vi "EnergyControlling.vi"() -> ()   [LabVIEW 2017]
uses:
  classes/DataCollector.lvclass
  classes/DataHandler.lvclass
  classes/SimulationParameter.lvclass
panel:
  in  "Controlling":T1={"Prioritization"=0, "Operating Mode"="", "Release Time "={"Start"=0.0, "Stop"=0.0}, "Activity"=TRUE, " Limitation"={"El. Power"=0.0, "Th. Power"=0.0}}
  in  "Field Elements":i32(listbox)
  in  "Management-Typs":u16(ring) items=["ManagementRandomData.vi", "ManagementRandomData2.vi"]
  in  "Stop":bool
  out "Control-Matrix-Overview":i32(listbox)=-1
  in  "application reference (local)":refnum<vi>
  out "Array":path[](array[path])
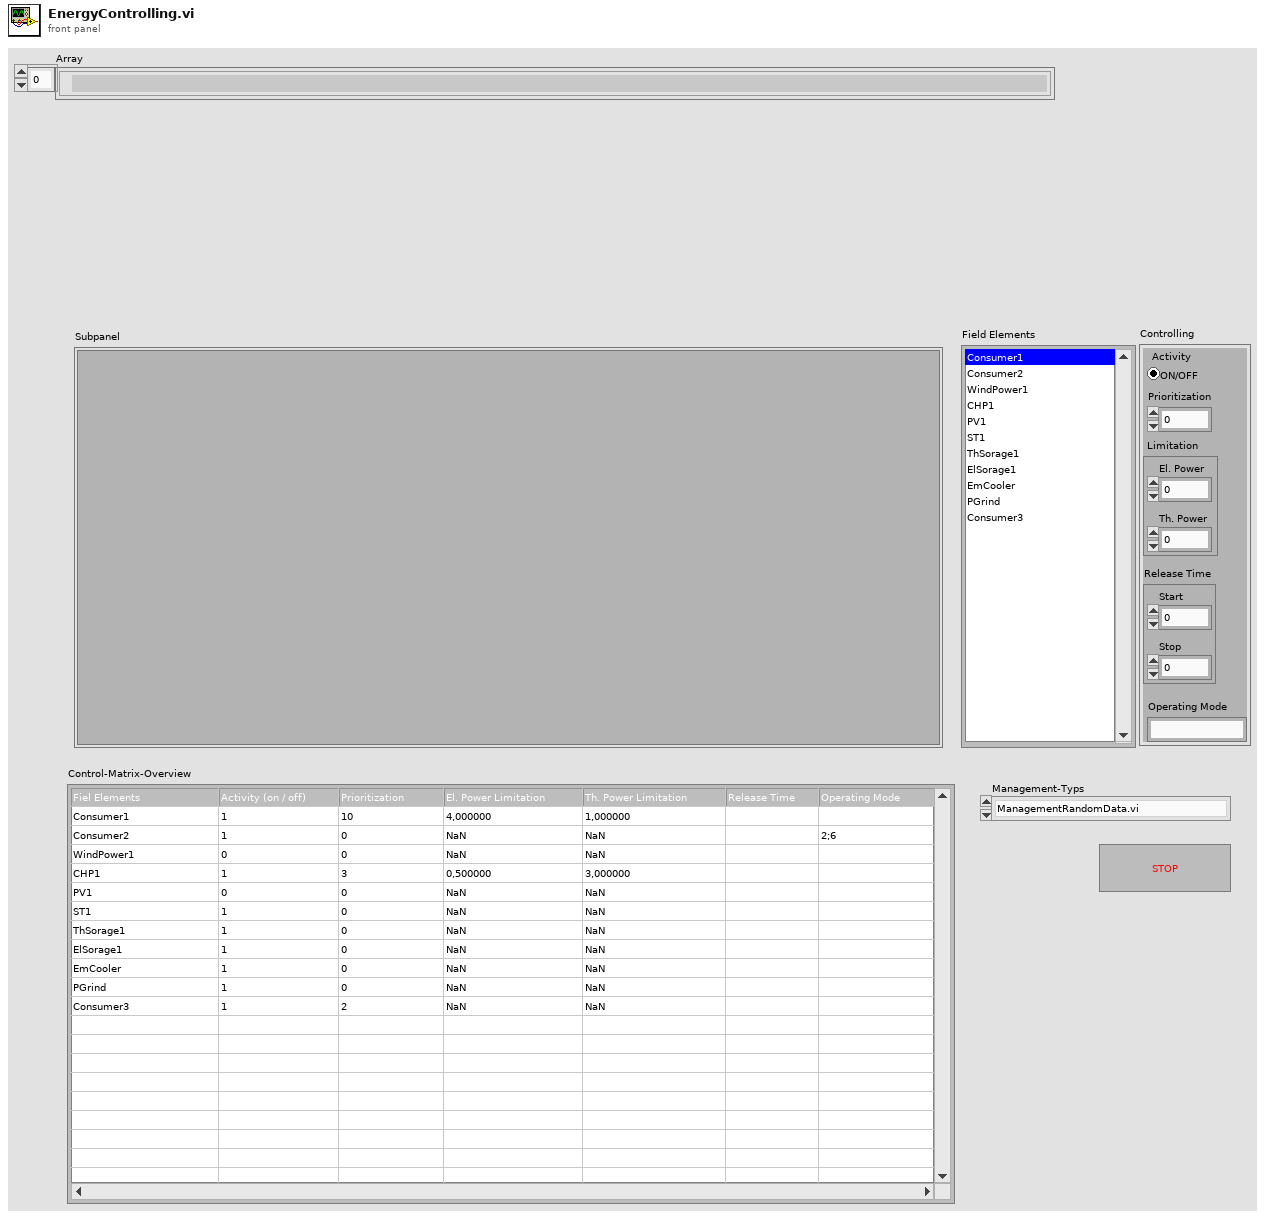
[diagram p1: front panel]
types:
  T1 = cluster{"Prioritization":i8, "Operating Mode":string, "Release Time ":cluster{"Start":dbl, "Stop":dbl}, "Activity":bool, " Limitation":cluster{"El. Power":dbl, "Th. Power":dbl}}
  T2 = cluster{"DataCollector out":refnum<class "DataCollector.lvclass">, "DataHandler out":refnum<class "DataHandler.lvclass">}
  T3 = cluster{"DataCollector":refnum<class "DataCollector.lvclass">, "DataHandling":refnum<class "DataHandler.lvclass">, "SimulationParameter":refnum<class "SimulationParameter.lvclass">}
  T4 = cluster{"DataCollector":refnum<class "DataCollector.lvclass">, "DataHandling":refnum<class "DataHandler.lvclass">}
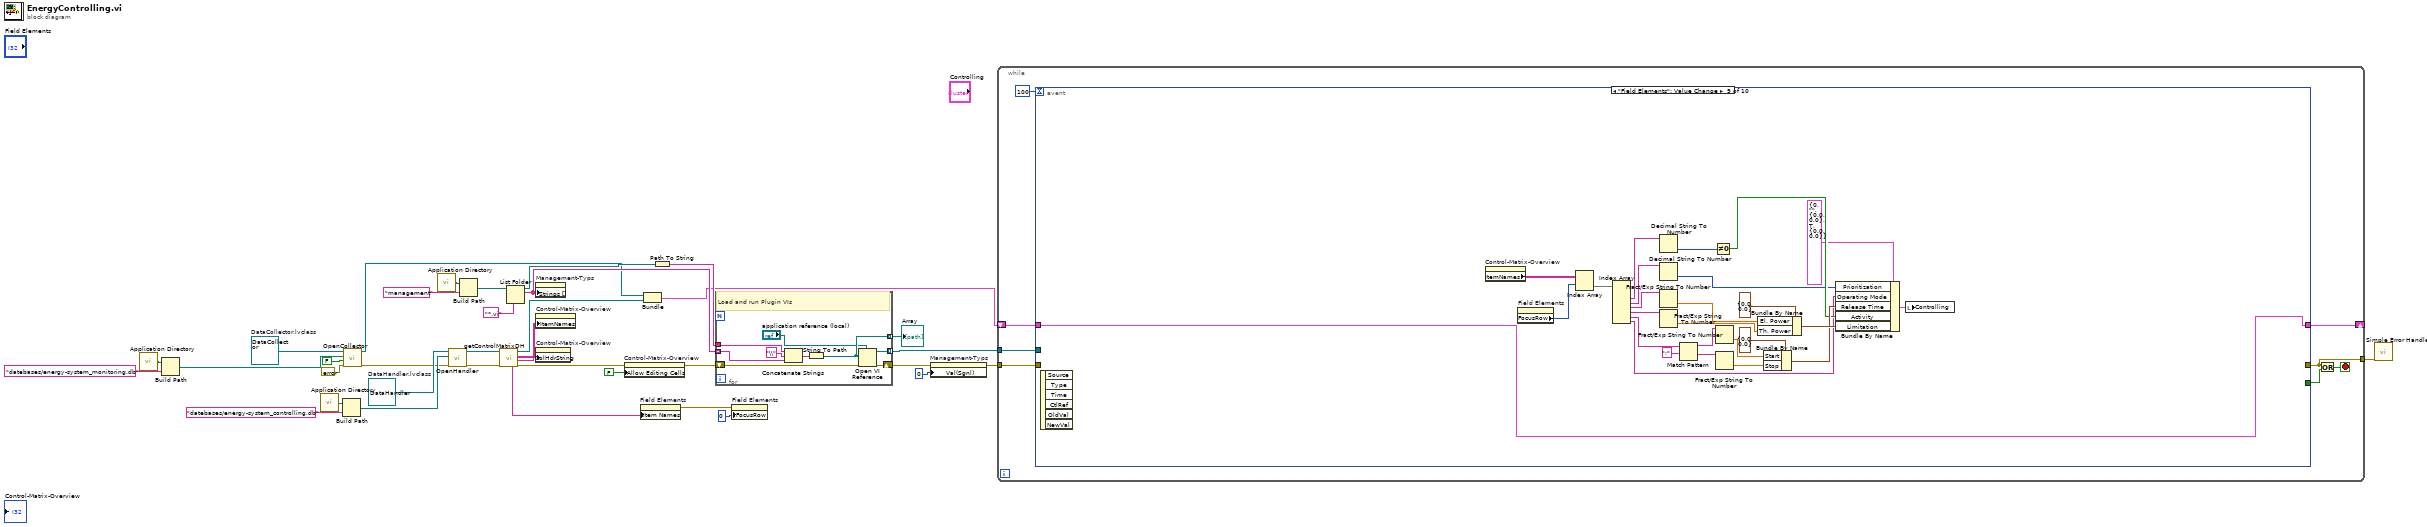
[diagram p0: block diagram]
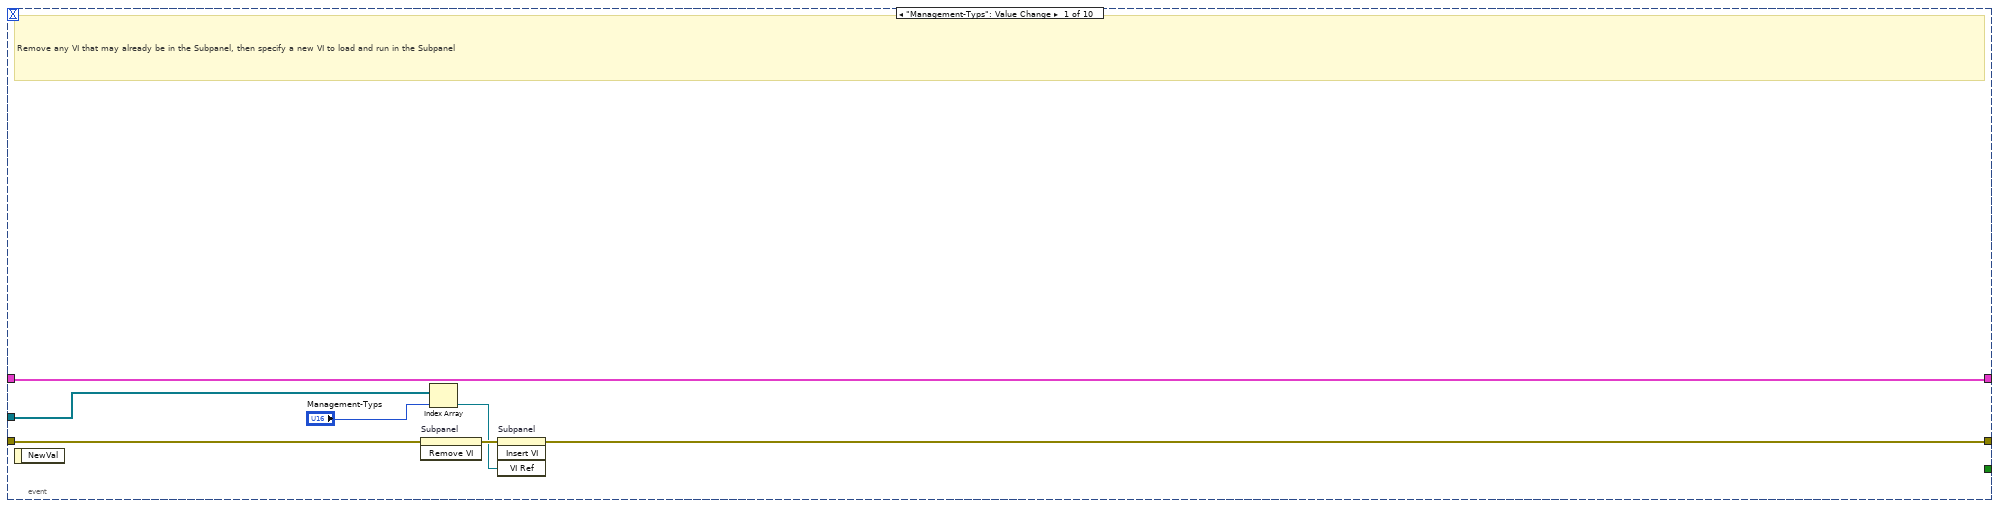
[diagram p2: hidden frame]
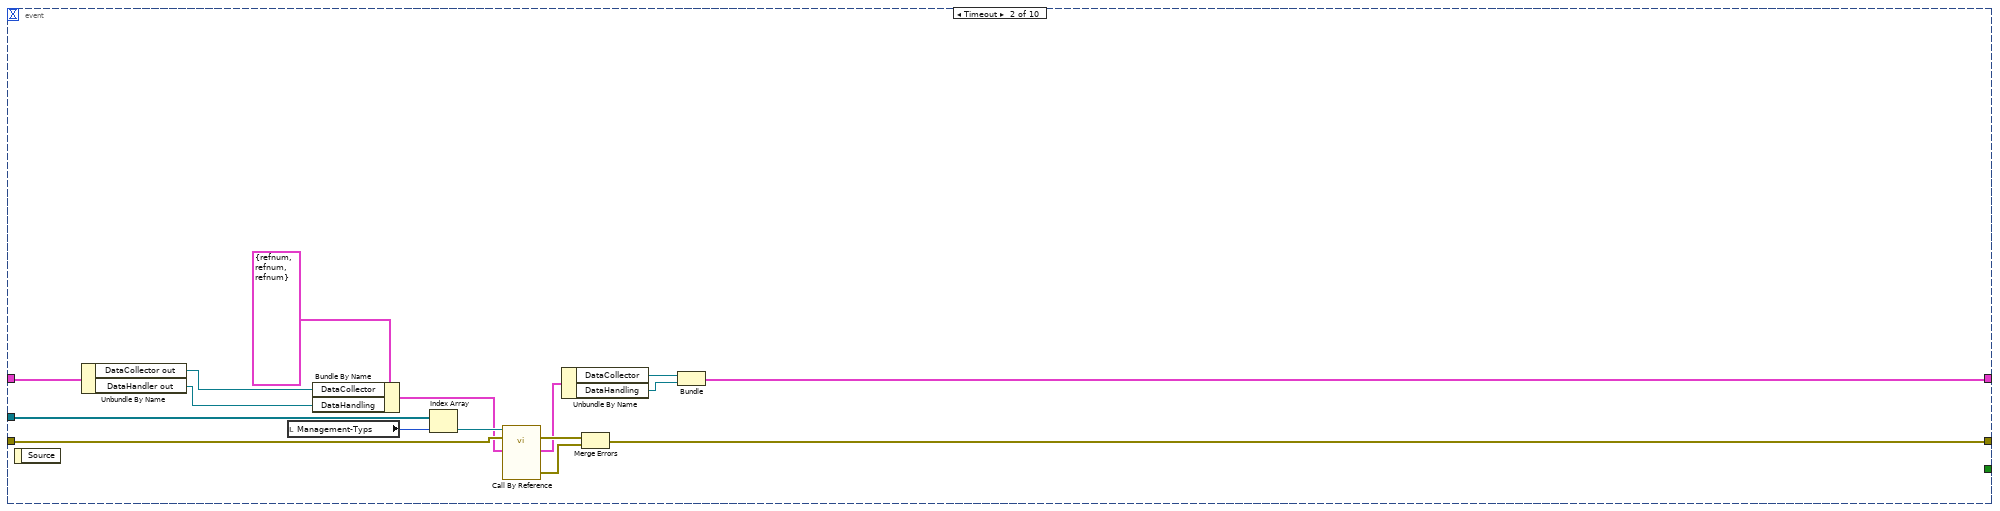
[diagram p3: hidden frame]
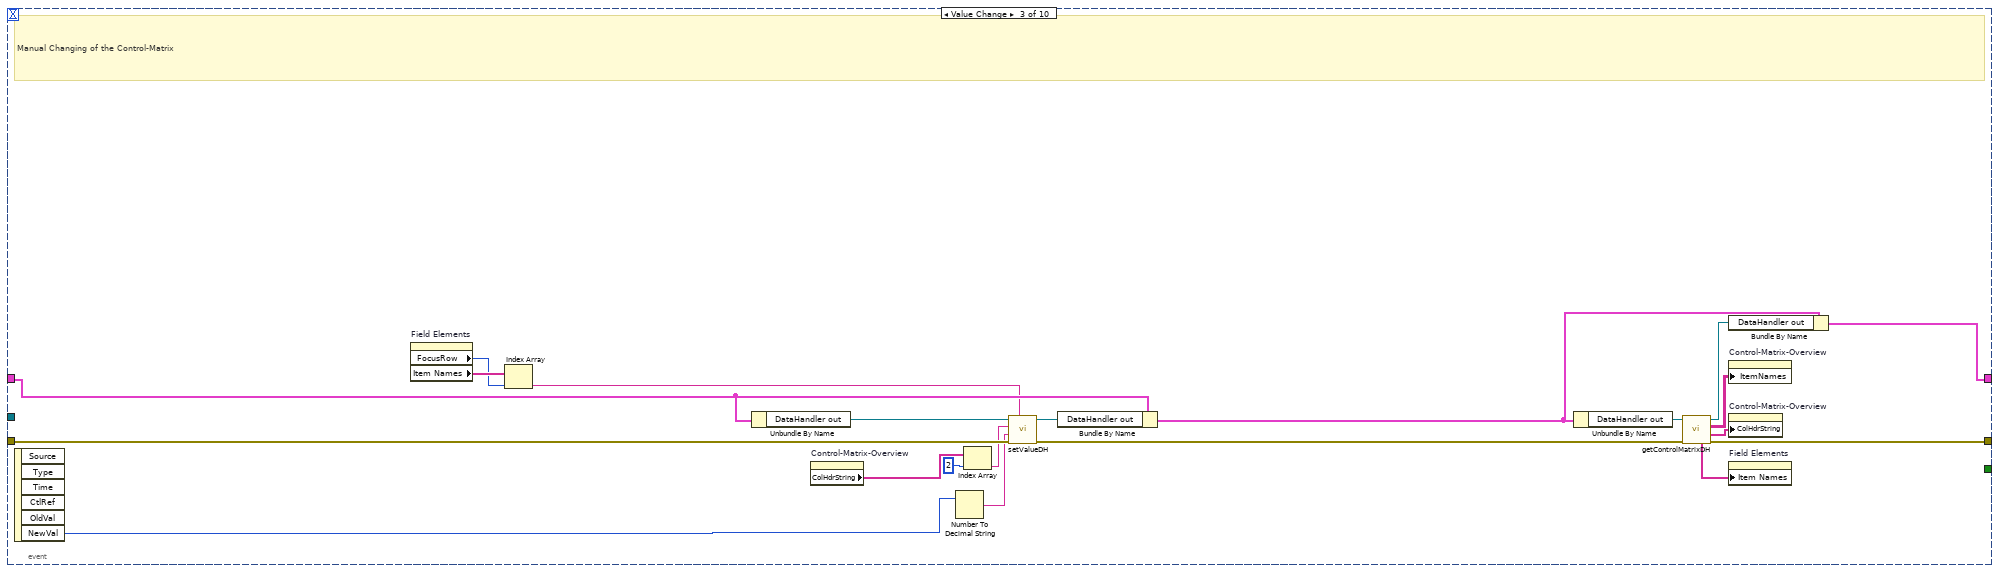
[diagram p4: hidden frame]
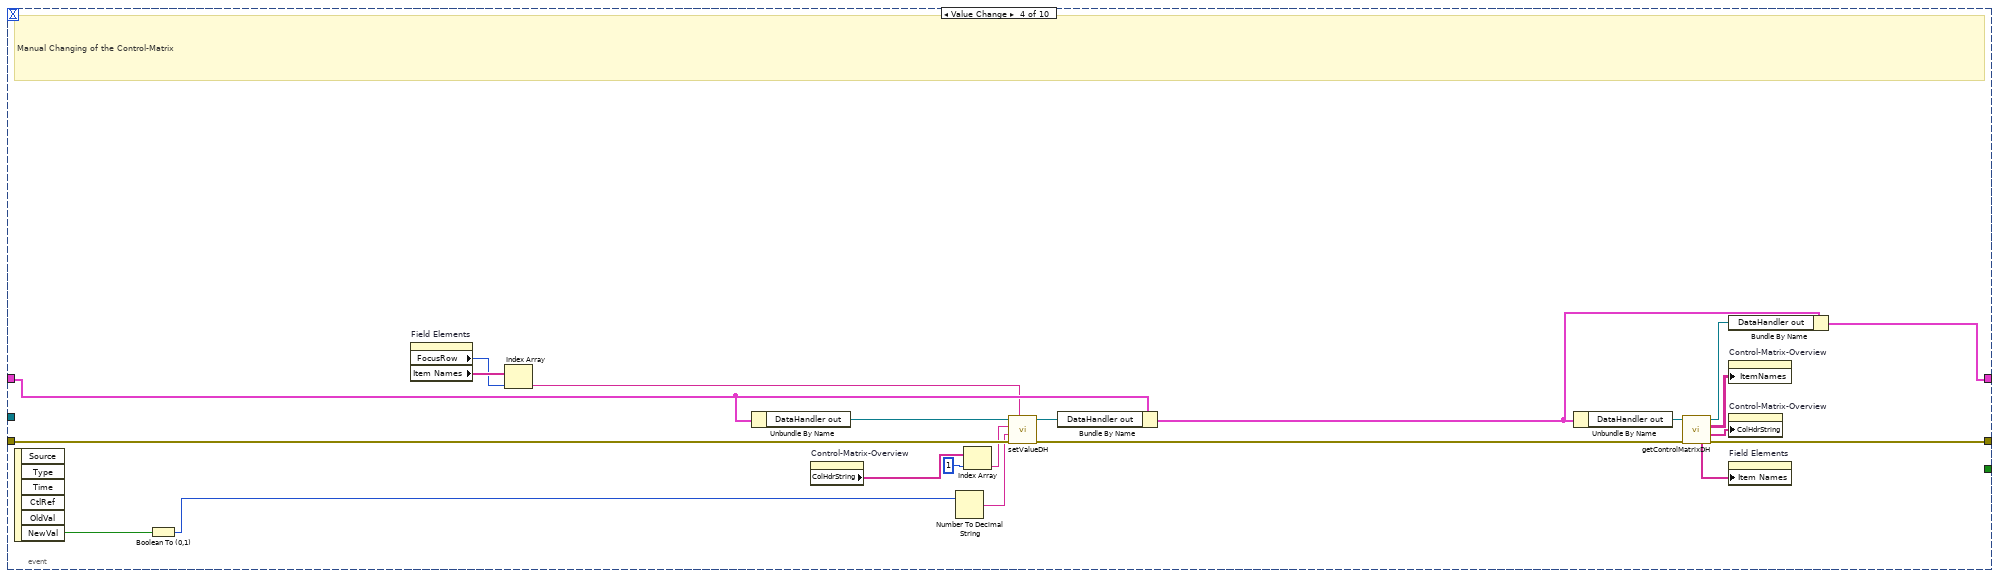
[diagram p5: hidden frame]
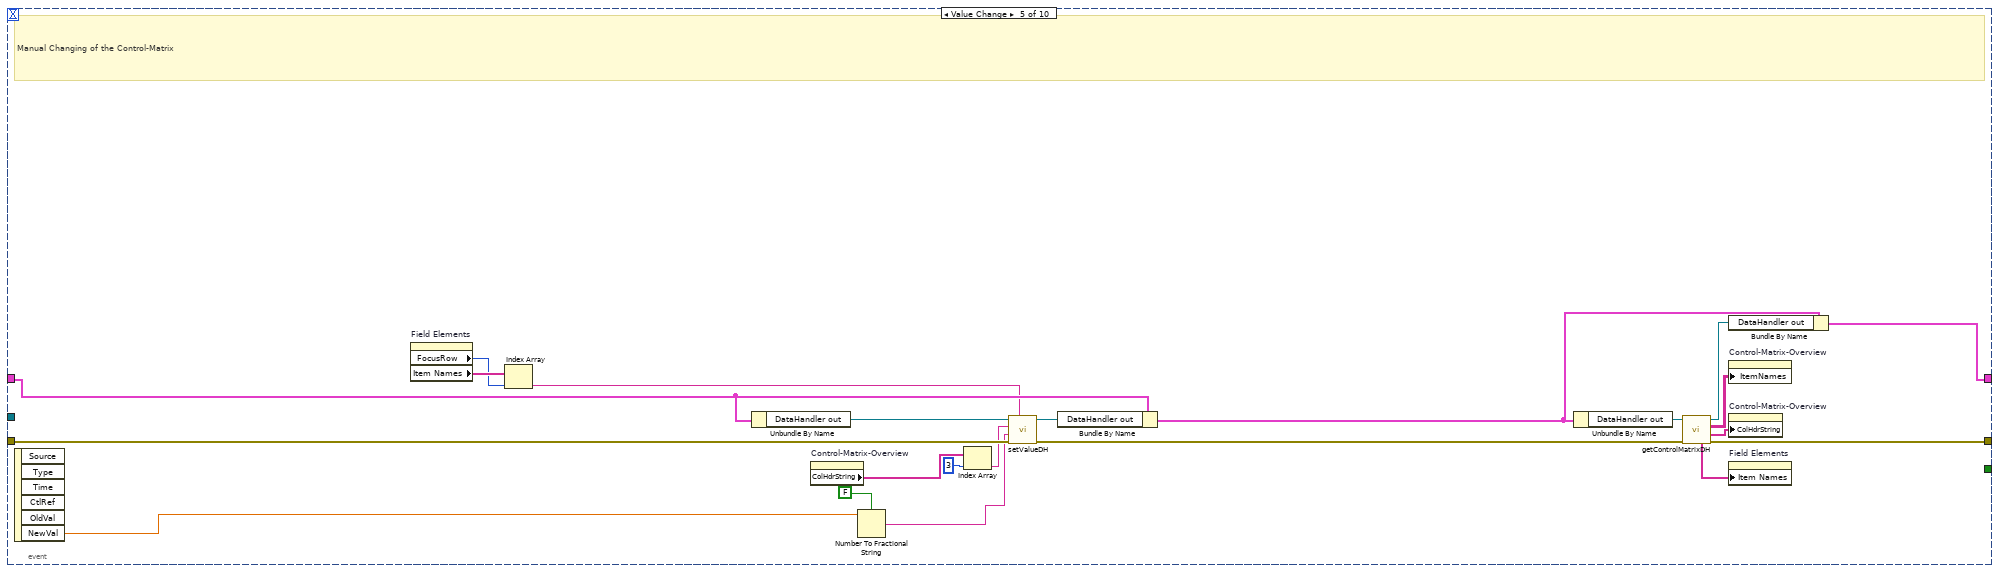
[diagram p6: hidden frame]
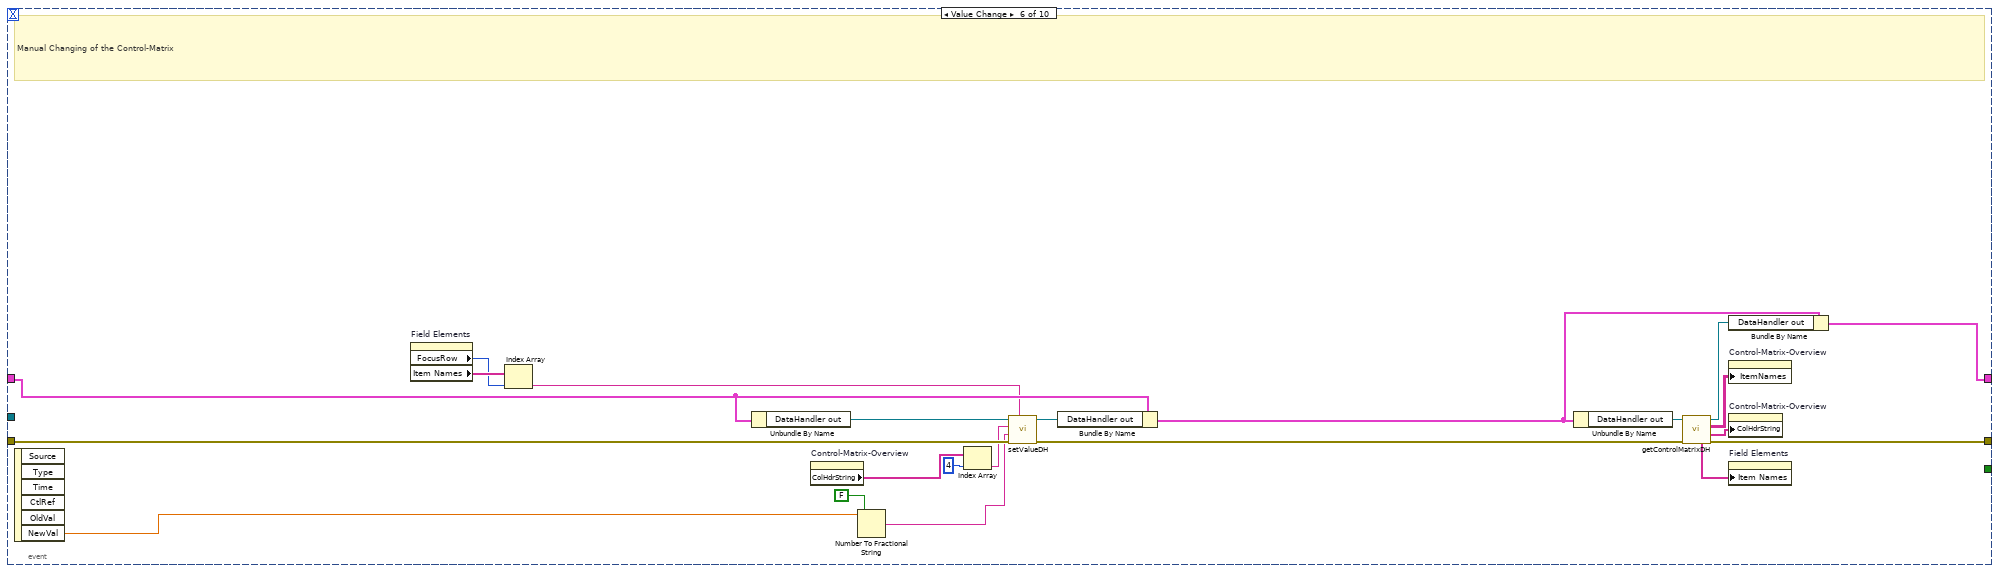
[diagram p7: hidden frame]
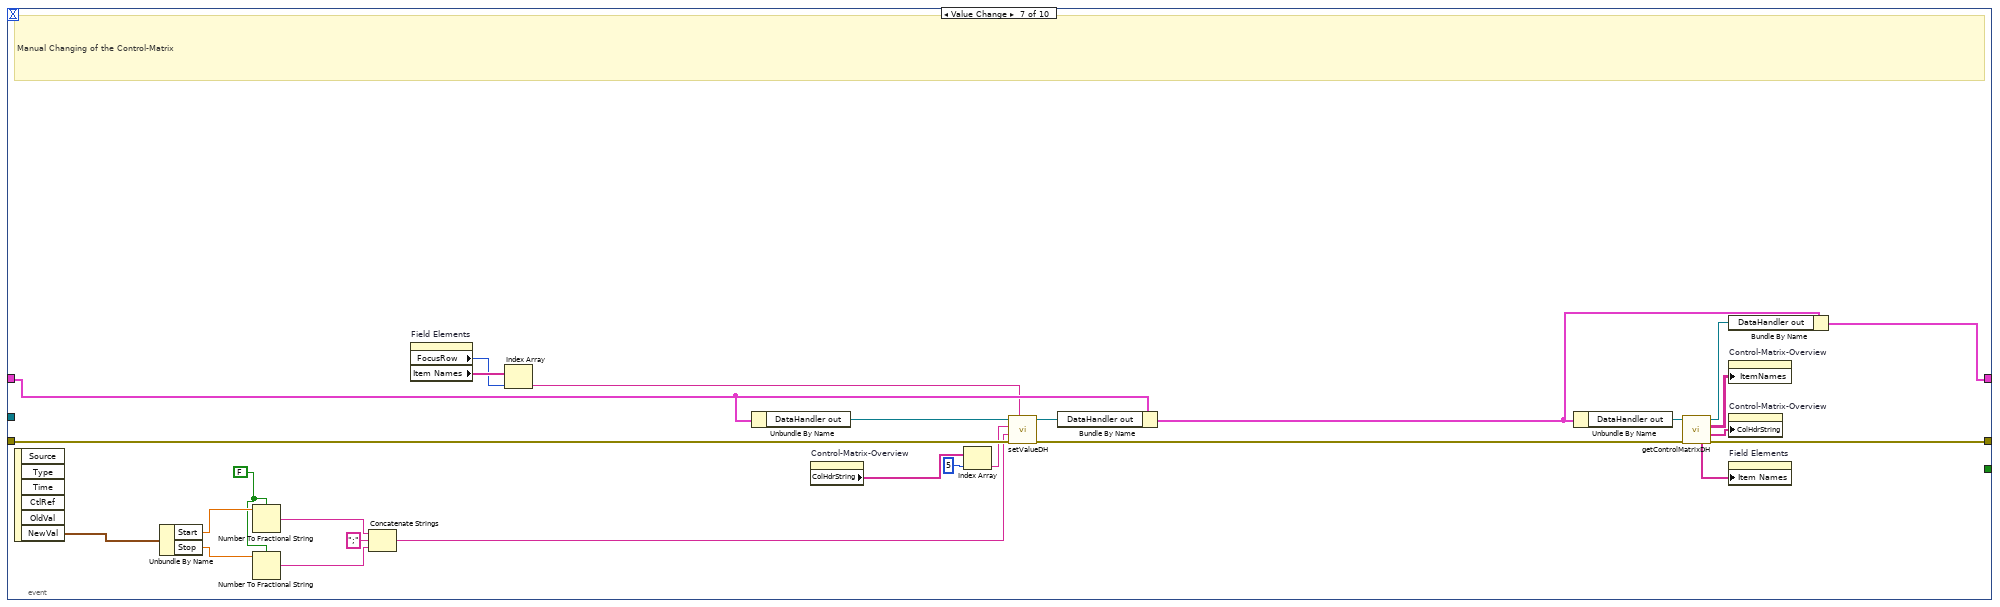
[diagram p8: hidden frame]
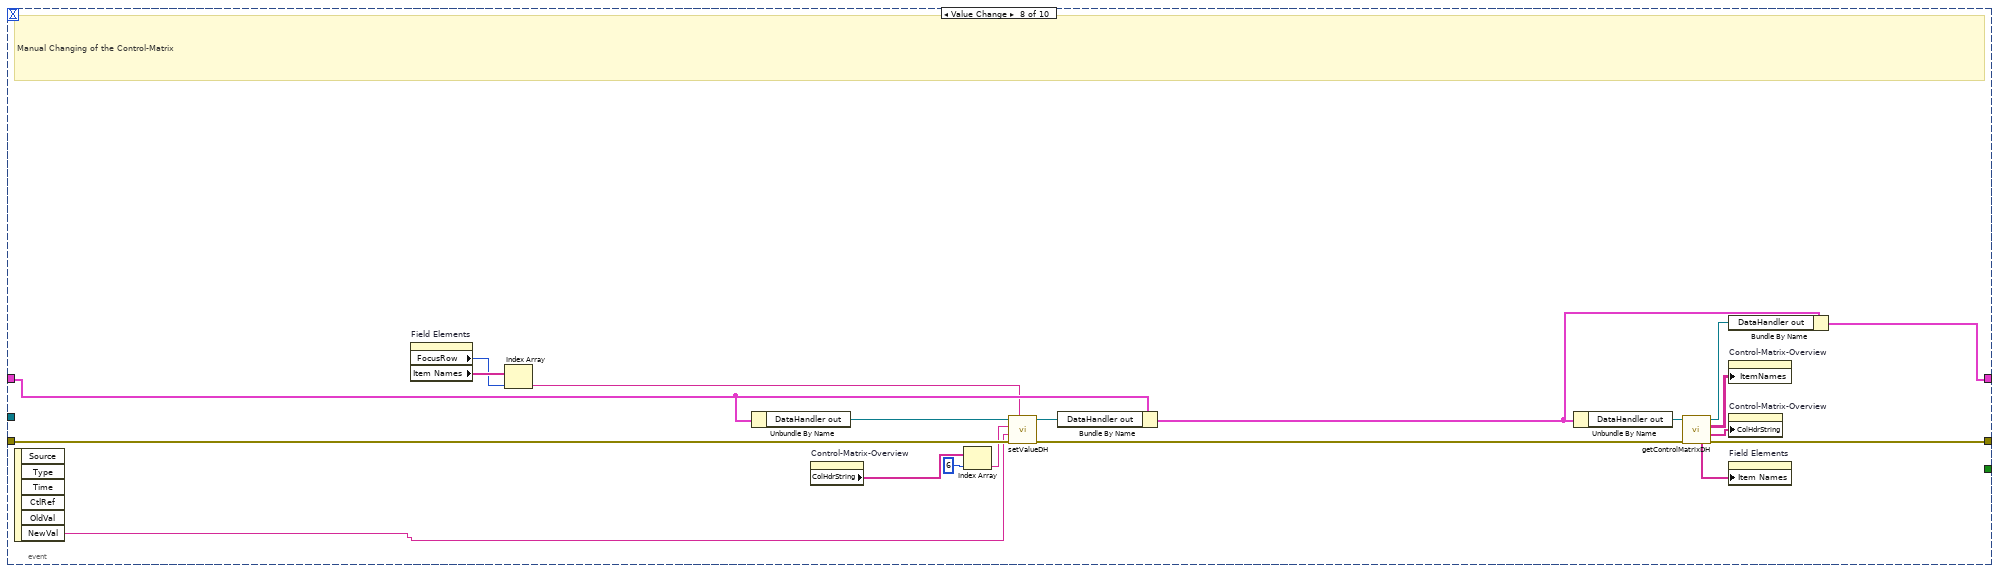
[diagram p9: hidden frame]
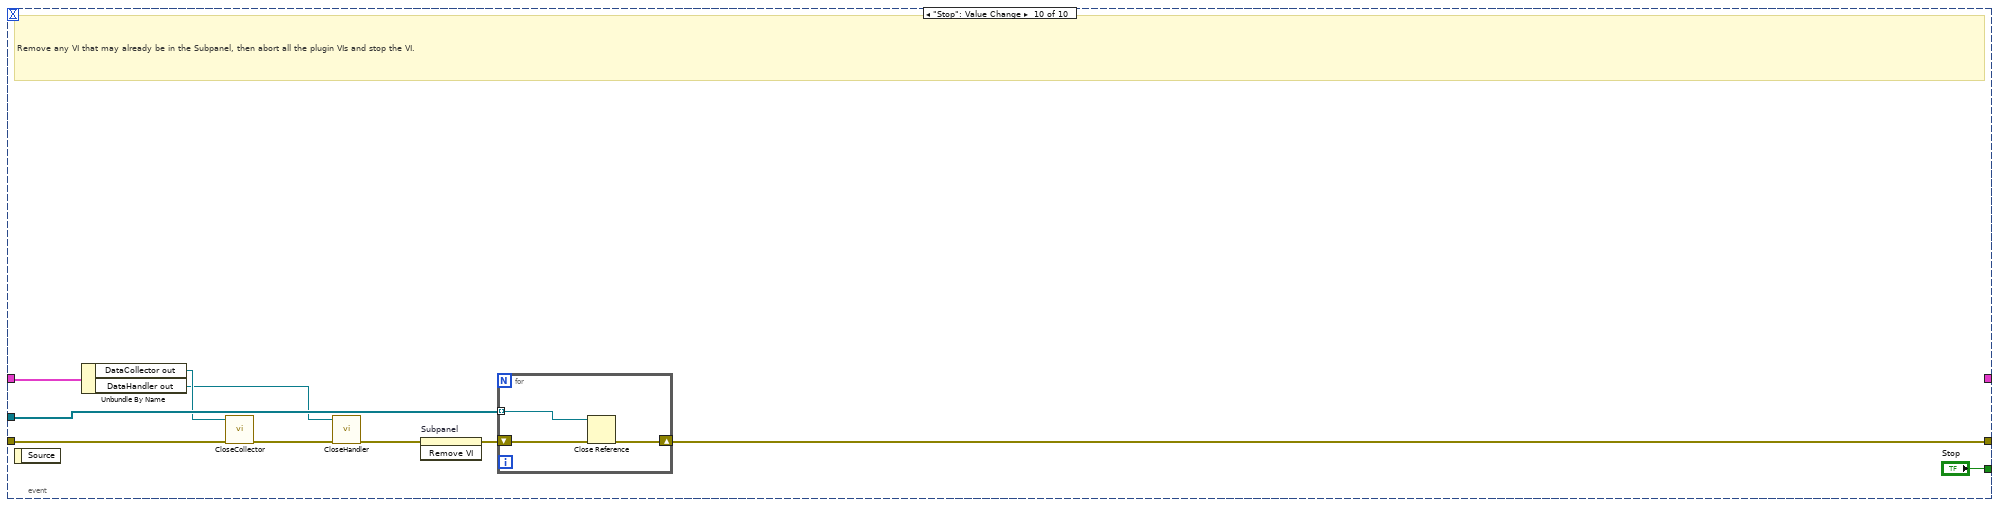
[diagram p10: hidden frame]
diagram:
  w19 = refnum<class "DataHandler.lvclass"> refnum  # DataHandler.lvclass
  w15 = refnum<class "DataCollector.lvclass"> refnum  # DataCollector.lvclass
  n1 = call <vilib>:"Application Directory.vi"() -> ("Application Directory"=w20:path)
  n2 = Build Path(base path=w20, name or relative path="datebases/energy-system_monitoring.db" ("Name oder relativer Pfad")) -> (appended path=w14:path)
  n3 = call <vilib>:"Application Directory.vi"() -> ("Application Directory"=w22:path)
  n4 = Build Path(base path=w22, name or relative path="datebases/energy-system_controlling.db" ("Name oder relativer Pfad")) -> (appended path=w21:path)
  n5 = call-dynamic "OpenCollector.vi"("error in (no error)"=errorcluster {"status"=FALSE, "code"=0, "source"=""} ("error constant"), "Ram?"=FALSE, "path to db monitoring"=w14, "DataCollector in"=w15) -> ("error out"=w6:errorcluster, "DataCollector out"=w13:refnum<class "DataCollector.lvclass">)  [unwired: 5 in, 1 out]
  n6 = call <vilib>:"Application Directory.vi"() -> ("Application Directory"=w27:path)
  n7 = call-dynamic "OpenHandler.vi"("error in (no error)"=w6, "path to db monitoring"=w21, "DataHandling in"=w19) -> ("error out"=w10:errorcluster, "DataHandling out"=w9:refnum<class "DataHandler.lvclass">)  [unwired: 7 in]
  n8 = Build Path(base path=w27, name or relative path="management" ("Name oder relativer Pfad")) -> (appended path=w28:path)
  n9 = call-dynamic "getControlMatrixDH.vi"("error in (no error)"=w10, "DataHandler in"=w9) -> ("error out"=w5:errorcluster, "List of ColHads"=w4:string[], "ControlParameterArrayMatrix"=w11:string[][], "DataHandler out"=w3:refnum<class "DataHandler.lvclass">, "Field Elements"=w8:string[])  [unwired: 5 in]
  n10 = List Folder(path=w28, pattern="*.vi") -> (path out=w32:path, filenames=w26:string[])  [unwired: 2 in, 2 out]
  n11 = property on="Management-Typs" class="Ring (strict)"("Strings []"=w26) -> ()  [unwired: 2 in, 2 out]
  n12 = property on="Control-Matrix-Overview" class="MCListbox (strict)"("ItemNames"=w11) -> ()  [unwired: 2 in, 2 out]
  n13 = property on="Control-Matrix-Overview" class="MCListbox (strict)"("ColHdrString"=w4) -> ()  [unwired: 2 in, 2 out]
  n14 = property on="Control-Matrix-Overview" class="MCListbox (strict)"(error in=w5, "Allow Editing Cells"=FALSE) -> (error out=w23:errorcluster)  [unwired: 1 in, 1 out]
  n15 = property on="Field Elements" class="LstBox (strict)"("Item Names"=w8) -> (error out=w1:errorcluster)  [unwired: 2 in, 1 out]
  n16 = Bundle("DataCollector out"=w13, "DataHandler out"=w3) -> (w12:T2)  [unwired: 1 in]
  n17 = Path To String(path=w32) -> (string=w31:string)
  n18 = for {
    tunnel: [w38] -> w25 mode=indexing
    shift-right: [w39] -> w34
    shift-left: w23 -> [w46]
    tunnel: w26 -> [w44] mode=indexing
    tunnel: w31 -> [w45]
    tunnel: [w42] -> w30 mode=indexing
    # "Load and run Plugin VIs"
    n19 = Concatenate Strings(w45, "\\" ("string"), w44) -> (w43:string)
    n20 = String To Path(string=w43) -> (path=w42:path)
    n21 = Open VI Reference(type specifier VI Refnum (for type only)="application reference (local)", vi path=w42, error in (no error)=w46) -> (vi reference=w38:refnum<vi>, error out=w39:errorcluster)  [unwired: 3 in]
  }
  "Array" <- w30
  n22 = property on="Field Elements" class="LstBox (strict)"(error in=w1, "FocusRow"=0 ("Focus Row")) -> ()  [unwired: 1 in, 2 out]
  n23 = property on="Management-Typs" class="Ring (strict)"(error in=w34, "Val(Sgnl)"=u16 0 ("Value (Signaling)")) -> (error out=w37:errorcluster)  [unwired: 1 in, 1 out]
  n24 = while {
    tunnel: w37 -> [w51]
    tunnel: [w52] -> w35
    tunnel: w25 -> [w49]
    shift-right: [w47] -> _
    shift-left: w12 -> [w48]
    stop <- w53 stop-if-true
    n25 = event shown="[8] \"Field Elements\": Value Change" {
      selector: _ -> [_ _ _ _ _ _ _ _ _ _]
      dyn-events: _ -> [_ _ _ _ _ _ _ _ _ _]
      timeout: 100 -> [_ _ _ _ _ _ _ _ _ _]
      tunnel: [_ _ _ _ _ _ _ _ _ "Stop"] -> w54
      tunnel: [w61 w71 w89 w111 w133 w155 w182 w202 _ w245] -> w52
      tunnel: w49 -> [w60 w76 _ _ _ _ _ _ _ w246]
      tunnel: w51 -> [w57 w74 w97 w119 w141 w163 w190 w210 _ w239]
      tunnel: w48 -> [w55 w69 w98 w120 w142 w164 w191 w211 w212 w240]
      tunnel: [w55 w62 w86 w108 w130 w152 w179 w199 w212 _] -> w47
      event "Management-Typs": Value Change {
        # "Remove any VI that may already be in the Subpanel, then specify a new VI to load and run in the Subpanel"
        n26 = event-data() -> ()  [unwired: 1 in, 1 out]
        n27 = invoke on="Subpanel" class="SubPnl" method="Remove VI"(error in=w57) -> (error out=w59:errorcluster)  [unwired: 2 in, 2 out]
        n28 = Index Array(array=w60, index="Management-Typs") -> (element=w58:refnum<vi>)
        n29 = invoke on="Subpanel" class="SubPnl" method="Insert VI"(error in=w59, "VI Ref"=w58) -> (error out=w61:errorcluster)  [unwired: 2 in, 3 out]
      }
      event Timeout {
        n30 = event-data() -> ()  [unwired: 1 in, 1 out]
        n31 = Unbundle By Name(w69) -> ("DataCollector out"=w67:refnum<class "DataCollector.lvclass">, "DataHandler out"=w68:refnum<class "DataHandler.lvclass">)
        n32 = local read "Management-Typs"() -> (w77:u16)
        n33 = Bundle By Name(cluster=T3 {"DataCollector"=refnum, "DataHandling"=refnum, "SimulationParameter"=refnum} ("DataFlowIN"), "DataCollector"=w67, "DataHandling"=w68) -> (w66:T3)
        n34 = Index Array(array=w76, index=w77) -> (element=w75:refnum<vi>)
        n35 = call-by-ref "?"(reference=w75, error in=w74, "DataFlowIN"=w66) -> (error out=w73:errorcluster, 0:"error out"=w72:errorcluster, "DataFlowOUT"=w65:T3)  [unwired: 9 in, 1 out]
        n36 = Unbundle By Name(w65) -> ("DataCollector"=w64:refnum<class "DataCollector.lvclass">, "DataHandling"=w63:refnum<class "DataHandler.lvclass">)
        n37 = Merge Errors(w73, w72) -> (w71:errorcluster)
        n38 = Bundle("DataCollector"=w64, "DataHandling"=w63) -> (w62:T4)  [unwired: 1 in]
      }
      event "Controlling.Prioritization": Value Change {
        # "Manual Changing of the Control-Matrix"
        n39 = event-data() -> ("NewVal"=w78:i8)  [unwired: 1 in, 5 out]
        n40 = property on="Field Elements" class="LstBox (strict)"() -> ("FocusRow"=w95:i32, "Item Names"=w96:string[])  [unwired: 2 in, 2 out]
        n41 = Index Array(array=w96, index=w95) -> (element=w94:string)
        n42 = Unbundle By Name(w98) -> ("DataHandler out"=w84:refnum<class "DataHandler.lvclass">)
        n43 = property on="Control-Matrix-Overview" class="MCListbox (strict)"() -> ("ColHdrString"=w81:string[])  [unwired: 2 in, 2 out]
        n44 = Number To Decimal String(number=w78) -> (decimal integer string=w82:string)  [unwired: 1 in]
        n45 = Index Array(array=w81, index=2) -> (element=w79:string)
        n46 = call-dynamic "setValueDH.vi"("TableName"=w94, "error in (no error)"=w97, "Value"=w82, "ItemName"=w79, "DataHandler in"=w84) -> ("error out"=w90:errorcluster, "DataHandler out"=w83:refnum<class "DataHandler.lvclass">)  [unwired: 5 in]
        n47 = Bundle By Name(cluster=w98, "DataHandler out"=w83) -> (w85:T2)
        n48 = Unbundle By Name(w85) -> ("DataHandler out"=w88:refnum<class "DataHandler.lvclass">)
        n49 = call-dynamic "getControlMatrixDH.vi"("error in (no error)"=w90, "DataHandler in"=w88) -> ("error out"=w89:errorcluster, "List of ColHads"=w91:string[], "ControlParameterArrayMatrix"=w93:string[][], "DataHandler out"=w87:refnum<class "DataHandler.lvclass">, "Field Elements"=w92:string[])  [unwired: 5 in]
        n50 = Bundle By Name(cluster=w85, "DataHandler out"=w87) -> (w86:T2)
        n51 = property on="Control-Matrix-Overview" class="MCListbox (strict)"("ItemNames"=w93) -> ()  [unwired: 2 in, 2 out]
        n52 = property on="Control-Matrix-Overview" class="MCListbox (strict)"("ColHdrString"=w91) -> ()  [unwired: 2 in, 2 out]
        n53 = property on="Field Elements" class="LstBox (strict)"("Item Names"=w92) -> ()  [unwired: 2 in, 2 out]
      }
      event "Controlling.Activity": Value Change {
        # "Manual Changing of the Control-Matrix"
        n54 = event-data() -> ("NewVal"=w100:bool)  [unwired: 1 in, 5 out]
        n55 = Boolean To (0,1)(Boolean=w100) -> (0, 1=w99:i16)
        n56 = property on="Field Elements" class="LstBox (strict)"() -> ("FocusRow"=w117:i32, "Item Names"=w118:string[])  [unwired: 2 in, 2 out]
        n57 = Index Array(array=w118, index=w117) -> (element=w116:string)
        n58 = Unbundle By Name(w120) -> ("DataHandler out"=w106:refnum<class "DataHandler.lvclass">)
        n59 = property on="Control-Matrix-Overview" class="MCListbox (strict)"() -> ("ColHdrString"=w103:string[])  [unwired: 2 in, 2 out]
        n60 = Number To Decimal String(number=w99) -> (decimal integer string=w104:string)  [unwired: 1 in]
        n61 = Index Array(array=w103, index=1) -> (element=w101:string)
        n62 = call-dynamic "setValueDH.vi"("TableName"=w116, "error in (no error)"=w119, "Value"=w104, "ItemName"=w101, "DataHandler in"=w106) -> ("error out"=w112:errorcluster, "DataHandler out"=w105:refnum<class "DataHandler.lvclass">)  [unwired: 5 in]
        n63 = Bundle By Name(cluster=w120, "DataHandler out"=w105) -> (w107:T2)
        n64 = Unbundle By Name(w107) -> ("DataHandler out"=w110:refnum<class "DataHandler.lvclass">)
        n65 = call-dynamic "getControlMatrixDH.vi"("error in (no error)"=w112, "DataHandler in"=w110) -> ("error out"=w111:errorcluster, "List of ColHads"=w113:string[], "ControlParameterArrayMatrix"=w115:string[][], "DataHandler out"=w109:refnum<class "DataHandler.lvclass">, "Field Elements"=w114:string[])  [unwired: 5 in]
        n66 = Bundle By Name(cluster=w107, "DataHandler out"=w109) -> (w108:T2)
        n67 = property on="Control-Matrix-Overview" class="MCListbox (strict)"("ItemNames"=w115) -> ()  [unwired: 2 in, 2 out]
        n68 = property on="Control-Matrix-Overview" class="MCListbox (strict)"("ColHdrString"=w113) -> ()  [unwired: 2 in, 2 out]
        n69 = property on="Field Elements" class="LstBox (strict)"("Item Names"=w114) -> ()  [unwired: 2 in, 2 out]
      }
      event "Controlling.Limitation.El. Power": Value Change {
        # "Manual Changing of the Control-Matrix"
        n70 = event-data() -> ("NewVal"=w123:dbl)  [unwired: 1 in, 5 out]
        n71 = property on="Field Elements" class="LstBox (strict)"() -> ("FocusRow"=w139:i32, "Item Names"=w140:string[])  [unwired: 2 in, 2 out]
        n72 = Index Array(array=w140, index=w139) -> (element=w138:string)
        n73 = Unbundle By Name(w142) -> ("DataHandler out"=w128:refnum<class "DataHandler.lvclass">)
        n74 = property on="Control-Matrix-Overview" class="MCListbox (strict)"() -> ("ColHdrString"=w126:string[])  [unwired: 2 in, 2 out]
        n75 = Number To Fractional String(use system decimal point (T)=FALSE, number=w123) -> (F-format string=w122:string)  [unwired: 2 in]
        n76 = Index Array(array=w126, index=3) -> (element=w124:string)
        n77 = call-dynamic "setValueDH.vi"("TableName"=w138, "error in (no error)"=w141, "Value"=w122, "ItemName"=w124, "DataHandler in"=w128) -> ("error out"=w134:errorcluster, "DataHandler out"=w127:refnum<class "DataHandler.lvclass">)  [unwired: 5 in]
        n78 = Bundle By Name(cluster=w142, "DataHandler out"=w127) -> (w129:T2)
        n79 = Unbundle By Name(w129) -> ("DataHandler out"=w132:refnum<class "DataHandler.lvclass">)
        n80 = call-dynamic "getControlMatrixDH.vi"("error in (no error)"=w134, "DataHandler in"=w132) -> ("error out"=w133:errorcluster, "List of ColHads"=w135:string[], "ControlParameterArrayMatrix"=w137:string[][], "DataHandler out"=w131:refnum<class "DataHandler.lvclass">, "Field Elements"=w136:string[])  [unwired: 5 in]
        n81 = Bundle By Name(cluster=w129, "DataHandler out"=w131) -> (w130:T2)
        n82 = property on="Control-Matrix-Overview" class="MCListbox (strict)"("ItemNames"=w137) -> ()  [unwired: 2 in, 2 out]
        n83 = property on="Control-Matrix-Overview" class="MCListbox (strict)"("ColHdrString"=w135) -> ()  [unwired: 2 in, 2 out]
        n84 = property on="Field Elements" class="LstBox (strict)"("Item Names"=w136) -> ()  [unwired: 2 in, 2 out]
      }
      event "Controlling.Limitation.Th. Power": Value Change {
        # "Manual Changing of the Control-Matrix"
        n85 = event-data() -> ("NewVal"=w145:dbl)  [unwired: 1 in, 5 out]
        n86 = property on="Field Elements" class="LstBox (strict)"() -> ("FocusRow"=w161:i32, "Item Names"=w162:string[])  [unwired: 2 in, 2 out]
        n87 = Index Array(array=w162, index=w161) -> (element=w160:string)
        n88 = Unbundle By Name(w164) -> ("DataHandler out"=w150:refnum<class "DataHandler.lvclass">)
        n89 = property on="Control-Matrix-Overview" class="MCListbox (strict)"() -> ("ColHdrString"=w148:string[])  [unwired: 2 in, 2 out]
        n90 = Number To Fractional String(use system decimal point (T)=FALSE, number=w145) -> (F-format string=w144:string)  [unwired: 2 in]
        n91 = Index Array(array=w148, index=4) -> (element=w146:string)
        n92 = call-dynamic "setValueDH.vi"("TableName"=w160, "error in (no error)"=w163, "Value"=w144, "ItemName"=w146, "DataHandler in"=w150) -> ("error out"=w156:errorcluster, "DataHandler out"=w149:refnum<class "DataHandler.lvclass">)  [unwired: 5 in]
        n93 = Bundle By Name(cluster=w164, "DataHandler out"=w149) -> (w151:T2)
        n94 = Unbundle By Name(w151) -> ("DataHandler out"=w154:refnum<class "DataHandler.lvclass">)
        n95 = call-dynamic "getControlMatrixDH.vi"("error in (no error)"=w156, "DataHandler in"=w154) -> ("error out"=w155:errorcluster, "List of ColHads"=w157:string[], "ControlParameterArrayMatrix"=w159:string[][], "DataHandler out"=w153:refnum<class "DataHandler.lvclass">, "Field Elements"=w158:string[])  [unwired: 5 in]
        n96 = Bundle By Name(cluster=w151, "DataHandler out"=w153) -> (w152:T2)
        n97 = property on="Control-Matrix-Overview" class="MCListbox (strict)"("ItemNames"=w159) -> ()  [unwired: 2 in, 2 out]
        n98 = property on="Control-Matrix-Overview" class="MCListbox (strict)"("ColHdrString"=w157) -> ()  [unwired: 2 in, 2 out]
        n99 = property on="Field Elements" class="LstBox (strict)"("Item Names"=w158) -> ()  [unwired: 2 in, 2 out]
      }
      event "Controlling.Release Time": Value Change {
        w165 = FALSE ("use system decimal point (T)")
        # "Manual Changing of the Control-Matrix"
        n100 = event-data() -> ("NewVal"=w172:cluster{"Start":dbl, "Stop":dbl})  [unwired: 1 in, 5 out]
        n101 = Unbundle By Name(w172) -> ("Start"=w171:dbl, "Stop"=w170:dbl)
        n102 = Number To Fractional String(use system decimal point (T)=w165, number=w171) -> (F-format string=w169:string)  [unwired: 2 in]
        n103 = Number To Fractional String(use system decimal point (T)=w165, number=w170) -> (F-format string=w168:string)  [unwired: 2 in]
        n104 = Concatenate Strings(w169, ";" ("string"), w168) -> (w166:string)
        n105 = property on="Field Elements" class="LstBox (strict)"() -> ("FocusRow"=w188:i32, "Item Names"=w189:string[])  [unwired: 2 in, 2 out]
        n106 = Index Array(array=w189, index=w188) -> (element=w187:string)
        n107 = Unbundle By Name(w191) -> ("DataHandler out"=w177:refnum<class "DataHandler.lvclass">)
        n108 = property on="Control-Matrix-Overview" class="MCListbox (strict)"() -> ("ColHdrString"=w175:string[])  [unwired: 2 in, 2 out]
        n109 = Index Array(array=w175, index=5) -> (element=w173:string)
        n110 = call-dynamic "setValueDH.vi"("TableName"=w187, "error in (no error)"=w190, "Value"=w166, "ItemName"=w173, "DataHandler in"=w177) -> ("error out"=w183:errorcluster, "DataHandler out"=w176:refnum<class "DataHandler.lvclass">)  [unwired: 5 in]
        n111 = Bundle By Name(cluster=w191, "DataHandler out"=w176) -> (w178:T2)
        n112 = Unbundle By Name(w178) -> ("DataHandler out"=w181:refnum<class "DataHandler.lvclass">)
        n113 = call-dynamic "getControlMatrixDH.vi"("error in (no error)"=w183, "DataHandler in"=w181) -> ("error out"=w182:errorcluster, "List of ColHads"=w184:string[], "ControlParameterArrayMatrix"=w186:string[][], "DataHandler out"=w180:refnum<class "DataHandler.lvclass">, "Field Elements"=w185:string[])  [unwired: 5 in]
        n114 = Bundle By Name(cluster=w178, "DataHandler out"=w180) -> (w179:T2)
        n115 = property on="Control-Matrix-Overview" class="MCListbox (strict)"("ItemNames"=w186) -> ()  [unwired: 2 in, 2 out]
        n116 = property on="Control-Matrix-Overview" class="MCListbox (strict)"("ColHdrString"=w184) -> ()  [unwired: 2 in, 2 out]
        n117 = property on="Field Elements" class="LstBox (strict)"("Item Names"=w185) -> ()  [unwired: 2 in, 2 out]
      }
      event "Controlling.Operating Mode": Value Change {
        # "Manual Changing of the Control-Matrix"
        n118 = event-data() -> ("NewVal"=w192:string)  [unwired: 1 in, 5 out]
        n119 = property on="Field Elements" class="LstBox (strict)"() -> ("FocusRow"=w208:i32, "Item Names"=w209:string[])  [unwired: 2 in, 2 out]
        n120 = Index Array(array=w209, index=w208) -> (element=w207:string)
        n121 = Unbundle By Name(w211) -> ("DataHandler out"=w197:refnum<class "DataHandler.lvclass">)
        n122 = property on="Control-Matrix-Overview" class="MCListbox (strict)"() -> ("ColHdrString"=w195:string[])  [unwired: 2 in, 2 out]
        n123 = Index Array(array=w195, index=6) -> (element=w193:string)
        n124 = call-dynamic "setValueDH.vi"("TableName"=w207, "error in (no error)"=w210, "Value"=w192, "ItemName"=w193, "DataHandler in"=w197) -> ("error out"=w203:errorcluster, "DataHandler out"=w196:refnum<class "DataHandler.lvclass">)  [unwired: 5 in]
        n125 = Bundle By Name(cluster=w211, "DataHandler out"=w196) -> (w198:T2)
        n126 = Unbundle By Name(w198) -> ("DataHandler out"=w201:refnum<class "DataHandler.lvclass">)
        n127 = call-dynamic "getControlMatrixDH.vi"("error in (no error)"=w203, "DataHandler in"=w201) -> ("error out"=w202:errorcluster, "List of ColHads"=w204:string[], "ControlParameterArrayMatrix"=w206:string[][], "DataHandler out"=w200:refnum<class "DataHandler.lvclass">, "Field Elements"=w205:string[])  [unwired: 5 in]
        n128 = Bundle By Name(cluster=w198, "DataHandler out"=w200) -> (w199:T2)
        n129 = property on="Control-Matrix-Overview" class="MCListbox (strict)"("ItemNames"=w206) -> ()  [unwired: 2 in, 2 out]
        n130 = property on="Control-Matrix-Overview" class="MCListbox (strict)"("ColHdrString"=w204) -> ()  [unwired: 2 in, 2 out]
        n131 = property on="Field Elements" class="LstBox (strict)"("Item Names"=w205) -> ()  [unwired: 2 in, 2 out]
      }
      event "Field Elements": Value Change {
        n132 = event-data() -> ()  [unwired: 1 in, 6 out]
        n133 = property on="Control-Matrix-Overview" class="MCListbox (strict)"() -> ("ItemNames"=w236:string[][])  [unwired: 2 in, 2 out]
        n134 = property on="Field Elements" class="LstBox (strict)"() -> ("FocusRow"=w237:i32)  [unwired: 2 in, 2 out]
        n135 = Index Array(array=w236, index (row)=w237) -> (element=w235:string[])  [unwired: 1 in]
        n136 = Index Array(array=w235) -> (element #2=w231:string, element #3=w229:string, element #4=w226:string, element #5=w223:string, element #6=w221:string, element #7=w222:string)  [unwired: 7 in, 1 out]
        n137 = Decimal String To Number(string=w231) -> (number=w227:i32)  [unwired: 2 in, 1 out]
        n138 = Decimal String To Number(string=w229) -> (number=w228:i32)  [unwired: 2 in, 1 out]
        n139 = Fract/Exp String To Number(string=w226) -> (number=w225:dbl)  [unwired: 3 in, 1 out]
        n140 = Fract/Exp String To Number(string=w223) -> (number=w224:dbl)  [unwired: 3 in, 1 out]
        n141 = Match Pattern(string=w221, regular expression=";") -> (before substring=w220:string, after substring=w219:string)  [unwired: 1 in, 2 out]
        n142 = Not Equal To 0?(x=w227) -> (x != 0?=w230:bool)
        n143 = Fract/Exp String To Number(string=w220) -> (number=w217:dbl)  [unwired: 3 in, 1 out]
        n144 = Fract/Exp String To Number(string=w219) -> (number=w218:dbl)  [unwired: 3 in, 1 out]
        n145 = Bundle By Name(cluster=cluster{"El. Power":dbl, "Th. Power":dbl} {"El. Power"=0.0, "Th. Power"=0.0} ("Limitation"), "El. Power"=w225, "Th. Power"=w224) -> (w233:cluster{"El. Power":dbl, "Th. Power":dbl})
        n146 = Bundle By Name(cluster=cluster{"Start":dbl, "Stop":dbl} {"Start"=0.0, "Stop"=0.0} ("Release Time"), "Start"=w217, "Stop"=w218) -> (w232:cluster{"Start":dbl, "Stop":dbl})
        n147 = Bundle By Name(cluster=T1 {"Prioritization"=0, "Operating Mode"="", "Release Time "={"Start"=0.0, "Stop"=0.0}, "Activity"=TRUE, " Limitation"={"El. Power"=0.0, "Th. Power"=0.0}} ("Controlling"), "Prioritization"=w228, "Operating Mode"=w222, "Release Time"=w232, "Activity"=w230, "Limitation"=w233) -> (w234:T1)
        n148 = local write "Controlling"(w234) -> ()
      }
      event "Stop": Value Change {
        # "Remove any VI that may already be in the Subpanel, then abort all the plugin VIs and stop the VI."
        n149 = event-data() -> ()  [unwired: 1 in, 1 out]
        n150 = Unbundle By Name(w240) -> ("DataCollector out"=w243:refnum<class "DataCollector.lvclass">, "DataHandler out"=w242:refnum<class "DataHandler.lvclass">)
        n151 = call "CloseCollector.vi"("error in (no error)"=w239, "DataCollector in"=w243) -> ("error out"=w241:errorcluster)  [unwired: 8 in, 1 out]
        n152 = call-dynamic "CloseHandler.vi"("error in (no error)"=w241, "DataHandling in"=w242) -> ("error out"=w238:errorcluster)  [unwired: 8 in, 1 out]
        n153 = invoke on="Subpanel" class="SubPnl" method="Remove VI"(error in=w238) -> (error out=w247:errorcluster)  [unwired: 2 in, 2 out]
        n154 = for {
          shift-right: [w250] -> w245
          shift-left: w247 -> [w249]
          tunnel: w246 -> [w248] mode=indexing
          n155 = Close Reference(reference=w248, error in (no error)=w249) -> (error out=w250:errorcluster)
        }
      }
    }
    n156 = Or(x=w52, y=w54) -> (x .or. y?=w53:bool)
  }
  n157 = call <vilib>:"Simple Error Handler.vi"("error in (no error)"=w35) -> ()  [unwired: 4 in, 5 out]
